vi "校准记录.vi"(8 "error in (no error)":errorcluster, 9 "曲线模型":T1={"标液浓度1"=0.0, "测量吸光度1"=0.0, "样品1启用"=FALSE, "标液浓度2"=0.0, "测量吸光度2"=0.0, "样品2启用"=FALSE, "标液浓度3"=0.0, "测量吸光度3"=0.0, "样品3启用"=FALSE, "标液浓度4"=0.0, "测量吸光度4"=0.0, "样品4启用"=FALSE, "标液浓度5"=0.0, "测量吸光度5"=0.0, "样品5启用"=FALSE, "模型"=enum."线性", "精度"=4.0, "XY图"=[], "拟合公式"="", "r^2"=0.0, "标样一校准时间"=timestamp(0 s since 1904-01-01), "标样二校准时间"=timestamp(0 s since 1904-01-01), "标样三校准时间"=timestamp(0 s since 1904-01-01), "标样四校准时间"=timestamp(0 s since 1904-01-01), "标样五校准时间"=timestamp(0 s since 1904-01-01), "二次方程"={"c"=0.0, "x"=0.0, "x^2"=0.0}, "标定时间"=timestamp(0 s since 1904-01-01), "拟合公式 2"="", "r^2 2"=0.0} {"r^2 2" format="%.7f"; "标定时间" format="%<%m/%d/%y %H:%M:%S>T"; "标样五校准时间" format="%<%m/%d/%y %H:%M:%S>T"; "标样四校准时间" format="%<%m/%d/%y %H:%M:%S>T"; "标样三校准时间" format="%<%m/%d/%y %H:%M:%S>T"; "标样二校准时间" format="%<%m/%d/%y %H:%M:%S>T"; "标样一校准时间" format="%<%m/%d/%y %H:%M:%S>T"; "r^2" format="%.7f"; "测量吸光度5" format="%#.6f"; "测量吸光度4" format="%#.6f"; "测量吸光度3" format="%#.6f"; "测量吸光度2" format="%#.6f"; "测量吸光度1" format="%#.6f"}, 10 "量程":enum16{"低量程", "高量程"}(ring), 11 "测量模式":string="所有测量模式") -> (0 "error out":errorcluster)   [LabVIEW 2016]
panel:
  out "结果字符串":string
  in  "data in":T2
  # "校准时间"
  # "标液浓度"
  # "吸光值显示"
  # "标液一"
  # "标液二"
  # "标液三"
  # "零点"
  # "跨度"
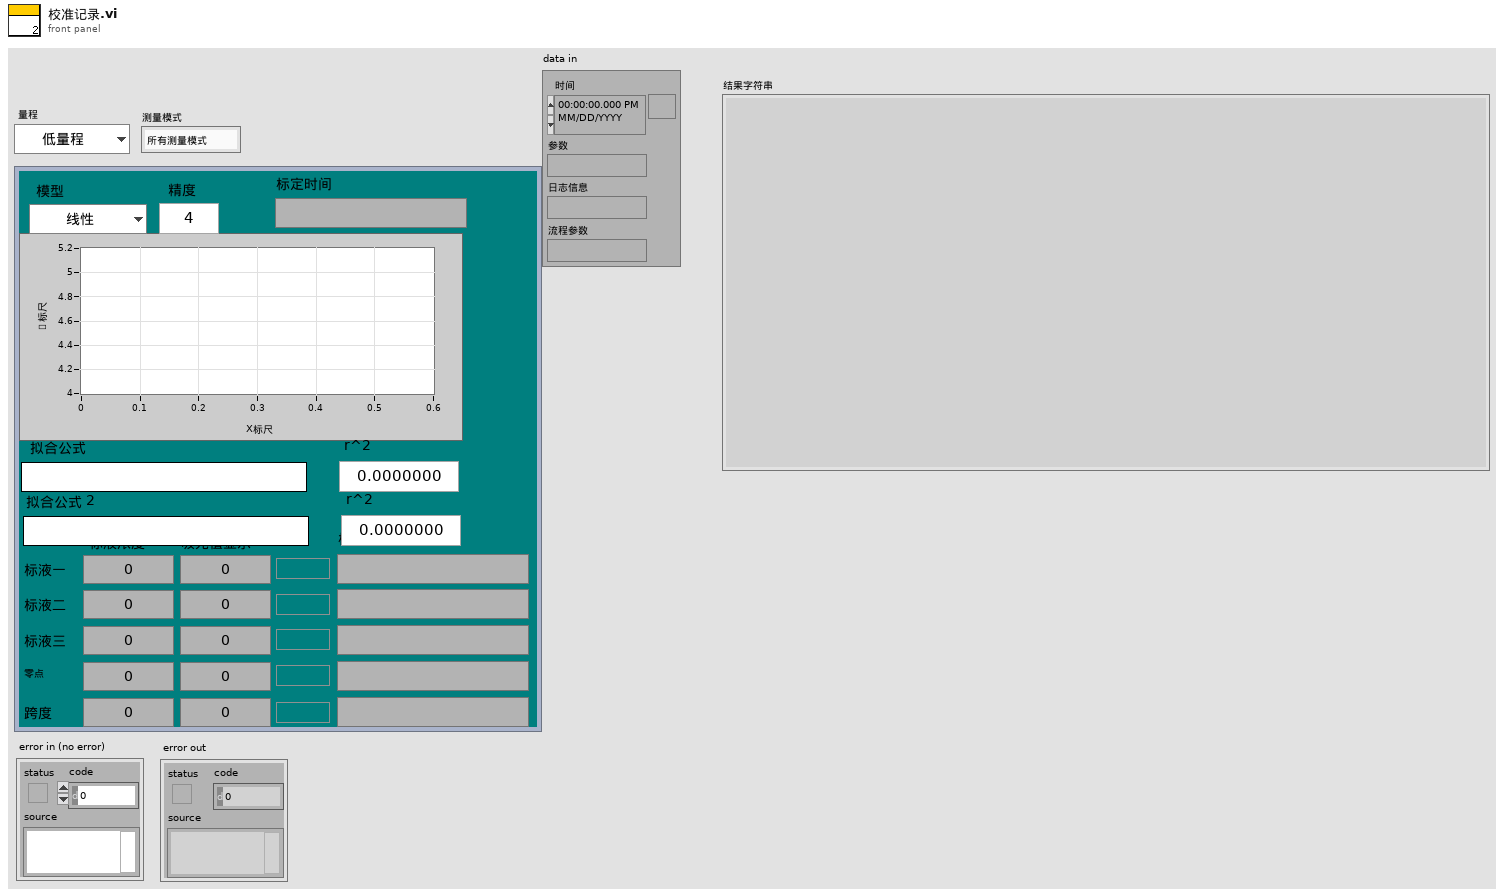
[diagram p1: front panel]
types:
  T1 = cluster{"标液浓度1":dbl, "测量吸光度1":dbl, "样品1启用":bool, "标液浓度2":dbl, "测量吸光度2":dbl, "样品2启用":bool, "标液浓度3":dbl, "测量吸光度3":dbl, "样品3启用":bool, "标液浓度4":dbl, "测量吸光度4":dbl, "样品4启用":bool, "标液浓度5":dbl, "测量吸光度5":dbl, "样品5启用":bool, "模型":enum32{"线性", "多项式", "折线"}, "精度":dbl, "XY图":cluster{"X Values":dbl[], "Y Values":dbl[]}[], "拟合公式":string, "r^2":dbl, "标样一校准时间":timestamp, "标样二校准时间":timestamp, "标样三校准时间":timestamp, "标样四校准时间":timestamp, "标样五校准时间":timestamp, "二次方程":cluster{"c":dbl, "x":dbl, "x^2":dbl}, "标定时间":timestamp, "拟合公式 2":string, "r^2 2":dbl}
  T2 = cluster{"时间":timestamp, "参数":string, "日志信息":string, "流程参数":string}
  T3 = cluster{"低标液1浓度":dbl, "低标液1信号值":dbl, "低标液1启用":u16, "低标液2浓度":dbl, "低标液2信号值":dbl, "低标液2启用":u16, "低标液3浓度":dbl, "低标液3信号值":dbl, "低标液3启用":u16, "低标液4浓度":dbl, "低标液4信号值":dbl, "低标液4启用":u16, "低标液5浓度":dbl, "低标液5信号值":dbl, "低标液5启用":u16, "高标液1浓度":dbl, "高标液1信号值":dbl, "高标液1启用":u16, "高标液2浓度":dbl, "高标液2信号值":dbl, "高标液2启用":u16, "高标液3浓度":dbl, "高标液3信号值":dbl, "高标液3启用":u16, "高标液4浓度":dbl, "高标液4信号值":dbl, "高标液4启用":u16, "高标液5浓度":dbl, "高标液5信号值":dbl, "高标液5启用":u16, "低斜率":dbl, "低截距":dbl, "低二次多项式系数":dbl, "低线性相关系数":dbl, "高斜率":dbl, "高截距":dbl, "高二次多项式系数":dbl, "高线性相关系数":dbl}
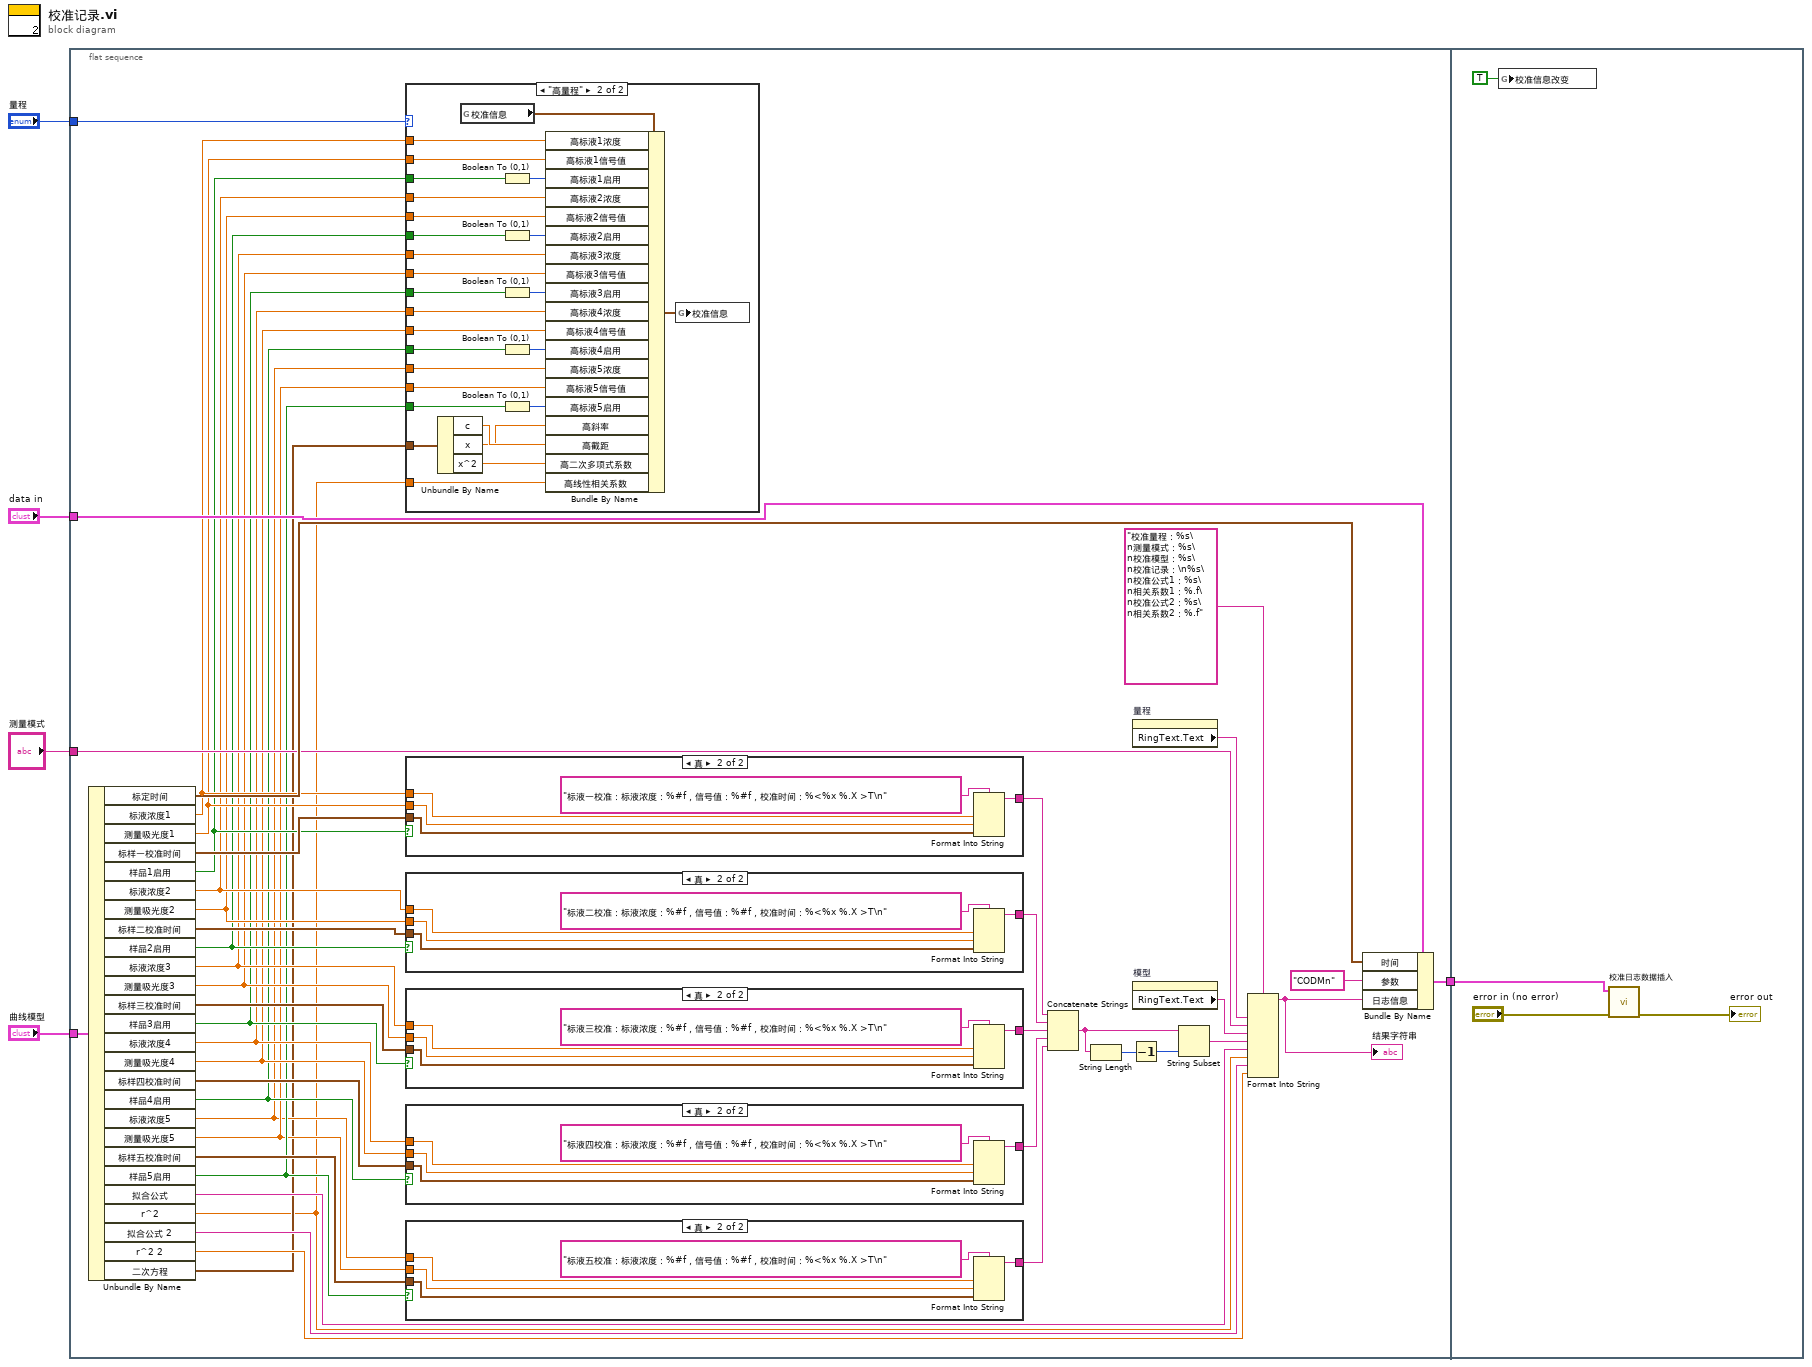
[diagram p0: block diagram]
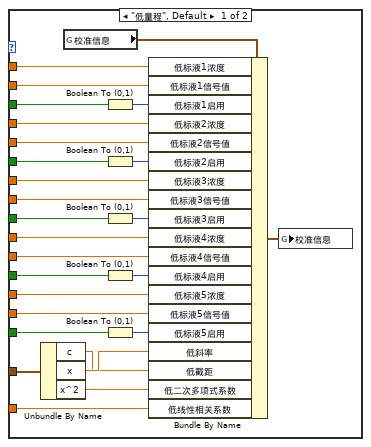
[diagram p2: hidden frame]
diagram:
  n1 = flat-sequence {
    tunnel: "量程" -> [w23]
    tunnel: "曲线模型" -> [w46]
    tunnel: "data in" -> [w50]
    tunnel: [w49] -> w2
    tunnel: "测量模式" -> [w24]
    tunnel: w2 -> [w131]
    frame #0 {
      n2 = Unbundle By Name(w46) -> ("标定时间"=w30:timestamp, "标液浓度1"=w22:dbl, "测量吸光度1"=w21:dbl, "标样一校准时间"=w45:timestamp, "样品1启用"=w20:bool, "标液浓度2"=w19:dbl, "测量吸光度2"=w18:dbl, "标样二校准时间"=w44:timestamp, "样品2启用"=w17:bool, "标液浓度3"=w16:dbl, "测量吸光度3"=w15:dbl, "标样三校准时间"=w43:timestamp, "样品3启用"=w14:bool, "标液浓度4"=w13:dbl, "测量吸光度4"=w12:dbl, "标样四校准时间"=w42:timestamp, "样品4启用"=w11:bool, "标液浓度5"=w8:dbl, "测量吸光度5"=w9:dbl, "标样五校准时间"=w41:timestamp, "样品5启用"=w10:bool, "拟合公式"=w35:string, "r^2"=w6:dbl, "拟合公式 2"=w28:string, "r^2 2"=w29:dbl, "二次方程"=w7:cluster{"c":dbl, "x":dbl, "x^2":dbl})
      n3 = case shown="\"高量程\"" w23 {
        tunnel: w22 -> [w75 w100]
        tunnel: w21 -> [w74 w99]
        tunnel: w20 -> [w72 w102]
        tunnel: w19 -> [w73 w98]
        tunnel: w18 -> [w70 w97]
        tunnel: w17 -> [w69 w96]
        tunnel: w16 -> [w67 w94]
        tunnel: w15 -> [w66 w93]
        tunnel: w14 -> [w65 w92]
        tunnel: w13 -> [w63 w87]
        tunnel: w12 -> [w62 w88]
        tunnel: w11 -> [w61 w90]
        tunnel: w10 -> [w56 w86]
        tunnel: w9 -> [w58 w84]
        tunnel: w8 -> [w59 w85]
        tunnel: w7 -> [w55 w82]
        tunnel: w6 -> [w51 w78]
        frame "低量程", Default {
          n4 = Unbundle By Name(w55) -> ("c"=w52:dbl, "x"=w53:dbl, "x^2"=w54:dbl)
          n5 = global read "挥发酚断电保存全局变量.vi" "校准信息"() -> (w77:T3)
          n6 = Boolean To (0,1)(Boolean=w72) -> (0, 1=w71:i16)
          n7 = Boolean To (0,1)(Boolean=w69) -> (0, 1=w68:i16)
          n8 = Boolean To (0,1)(Boolean=w65) -> (0, 1=w64:i16)
          n9 = Boolean To (0,1)(Boolean=w61) -> (0, 1=w60:i16)
          n10 = Boolean To (0,1)(Boolean=w56) -> (0, 1=w57:i16)
          n11 = Bundle By Name(cluster=w77, "低标液1浓度"=w75, "低标液1信号值"=w74, "低标液1启用"=w71, "低标液2浓度"=w73, "低标液2信号值"=w70, "低标液2启用"=w68, "低标液3浓度"=w67, "低标液3信号值"=w66, "低标液3启用"=w64, "低标液4浓度"=w63, "低标液4信号值"=w62, "低标液4启用"=w60, "低标液5浓度"=w59, "低标液5信号值"=w58, "低标液5启用"=w57, "低斜率"=w53, "低截距"=w52, "低二次多项式系数"=w54, "低线性相关系数"=w51) -> (w76:T3)
          n12 = global write "挥发酚断电保存全局变量.vi" "校准信息"(w76) -> ()
        }
        frame "高量程" {
          n13 = Unbundle By Name(w82) -> ("c"=w81:dbl, "x"=w80:dbl, "x^2"=w79:dbl)
          n14 = global read "挥发酚断电保存全局变量.vi" "校准信息"() -> (w104:T3)
          n15 = Boolean To (0,1)(Boolean=w102) -> (0, 1=w101:i16)
          n16 = Boolean To (0,1)(Boolean=w96) -> (0, 1=w95:i16)
          n17 = Boolean To (0,1)(Boolean=w92) -> (0, 1=w91:i16)
          n18 = Boolean To (0,1)(Boolean=w90) -> (0, 1=w89:i16)
          n19 = Boolean To (0,1)(Boolean=w86) -> (0, 1=w83:i16)
          n20 = Bundle By Name(cluster=w104, "高标液1浓度"=w100, "高标液1信号值"=w99, "高标液1启用"=w101, "高标液2浓度"=w98, "高标液2信号值"=w97, "高标液2启用"=w95, "高标液3浓度"=w94, "高标液3信号值"=w93, "高标液3启用"=w91, "高标液4浓度"=w87, "高标液4信号值"=w88, "高标液4启用"=w89, "高标液5浓度"=w85, "高标液5信号值"=w84, "高标液5启用"=w83, "高斜率"=w80, "高截距"=w81, "高二次多项式系数"=w79, "高线性相关系数"=w78) -> (w103:T3)
          n21 = global write "挥发酚断电保存全局变量.vi" "校准信息"(w103) -> ()
        }
      }
      n22 = case shown="真" w20 {
        tunnel: w22 -> [_ w128]
        tunnel: w21 -> [_ w127]
        tunnel: w45 -> [_ w126]
        tunnel: [_ w125] -> w40
        frame False {
        }
        frame True {
          n23 = Format Into String(format string="标液一校准：标液浓度：%#f，信号值：%#f，校准时间：%<%x %.X >T\n" ("格式字符串"), w128, w127, w126) -> (resulting string=w125:string)  [unwired: 2 in, 1 out]
        }
      }
      n24 = case shown="真" w17 {
        tunnel: w19 -> [_ w123]
        tunnel: w18 -> [_ w122]
        tunnel: w44 -> [_ w121]
        tunnel: [_ w120] -> w39
        frame False {
        }
        frame True {
          n25 = Format Into String(format string="标液二校准：标液浓度：%#f，信号值：%#f，校准时间：%<%x %.X >T\n" ("格式字符串"), w123, w122, w121) -> (resulting string=w120:string)  [unwired: 2 in, 1 out]
        }
      }
      n26 = case shown="真" w14 {
        tunnel: w16 -> [_ w118]
        tunnel: w15 -> [_ w117]
        tunnel: w43 -> [_ w116]
        tunnel: [_ w115] -> w38
        frame False {
        }
        frame True {
          n27 = Format Into String(format string="标液三校准：标液浓度：%#f，信号值：%#f，校准时间：%<%x %.X >T\n" ("格式字符串"), w118, w117, w116) -> (resulting string=w115:string)  [unwired: 2 in, 1 out]
        }
      }
      n28 = case shown="真" w11 {
        tunnel: w13 -> [_ w113]
        tunnel: w12 -> [_ w112]
        tunnel: w42 -> [_ w111]
        tunnel: [_ w110] -> w37
        frame False {
        }
        frame True {
          n29 = Format Into String(format string="标液四校准：标液浓度：%#f，信号值：%#f，校准时间：%<%x %.X >T\n" ("格式字符串"), w113, w112, w111) -> (resulting string=w110:string)  [unwired: 2 in, 1 out]
        }
      }
      n30 = case shown="真" w10 {
        tunnel: w8 -> [_ w108]
        tunnel: w9 -> [_ w107]
        tunnel: w41 -> [_ w106]
        tunnel: [_ w105] -> w36
        frame False {
        }
        frame True {
          n31 = Format Into String(format string="标液五校准：标液浓度：%#f，信号值：%#f，校准时间：%<%x %.X >T\n" ("格式字符串"), w108, w107, w106) -> (resulting string=w105:string)  [unwired: 2 in, 1 out]
        }
      }
      n32 = Concatenate Strings(w40, w39, w38, w37, w36) -> (w33:string)
      n33 = String Length(string=w33) -> (length=w32:i32)
      n34 = Decrement(x=w32) -> (x-1=w31:i32)
      n35 = property on="量程" class="Enum (严格)"() -> ("RingText.Text"=w25:string)  [unwired: 2 in, 2 out]
      n36 = property on="模型" class="Enum (严格)"() -> ("RingText.Text"=w27:string)  [unwired: 2 in, 2 out]
      n37 = String Subset(string=w33, length (rest)=w31) -> (substring=w34:string)  [unwired: 1 in]
      n38 = Format Into String(format string="校准量程：%s\n测量模式：%s\n校准模型：%s\n校准记录：\n%s\n校准公式1：%s\n相关系数1：%.f\n校准公式2：%s\n相关系数2：%.f" ("格式字符串"), w25, w24, w27, w34, w35, w6, w28, w29) -> (resulting string=w48:string)  [unwired: 2 in, 1 out]
      "结果字符串" <- w48
      n39 = Bundle By Name(cluster=w50, "时间"=w30, "参数"="CODMn", "日志信息"=w48) -> (w49:T2)
    }
    frame #1 {
      n40 = global write "挥发酚断电保存全局变量.vi" "校准信息改变"(TRUE ("关键参数改变")) -> ()
      n41 = call "校准日志数据插入.vi"("data"=w131, "错误输入（无错误）"="error in (no error)") -> ("错误输出"=→"error out":errorcluster)  [unwired: 8 in]
    }
  }
